vi "DHE_version.vi"(0 "fd in":i32, 5 "full":bool, 11 "error in (no error)":errorcluster) -> (4 "fd out":i32, 6 "version":string, 15 "error out":errorcluster)   [LabVIEW 2016]
doc: "This VI closes the I/O interface with the instrument."
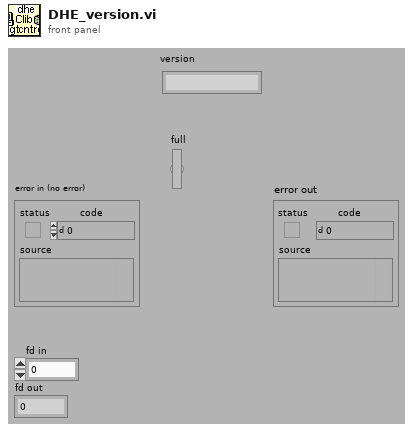
[diagram p1: front panel]
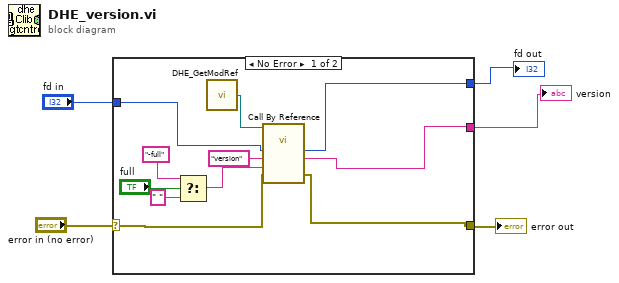
[diagram p0: block diagram]
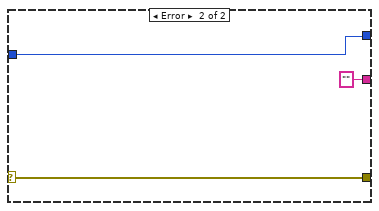
[diagram p2: hidden frame]
diagram:
  n1 = case shown="No Error" "error in (no error)" {
    selector: "error in (no error)" -> [w12 w19]
    tunnel: [w13 w19] -> w5
    tunnel: [w11 "" ("str result")] -> w1
    tunnel: "fd in" -> [w15 w18]
    tunnel: [w14 w18] -> w2
    frame No Error {
      n2 = Select(t="-full" ("function"), s="full", f=" ") -> (s? t:f=w6:string)
      n3 = call "DHE_GetModRef.vi"() -> ("DHE_ModRef"=w16:refnum<vi>)  [unwired: 9 out]
      n4 = call-by-ref "?"(reference=w16, "error in (no error)"=w12, "arguments"=w6, "function"="version", "fd in"=w15) -> ("error out"=w13:errorcluster, "str result"=w11:string, "fd out"=w14:i32)  [unwired: 5 in, 3 out]
    }
    frame Error {
    }
  }
  "error out" <- w5
  "version" <- w1
  "fd out" <- w2
